vi "URG-04LX-UG01 Change Baud Rate.vi"(8 "error in":errorcluster, 10 "Baud Rate":u32, 11 "VISA Refnum in":refnum<visa-resource-name>) -> (0 "error out":errorcluster, 3 "VISA Refnum out":refnum<visa-resource-name>)   [LabVIEW 2018]
doc: "Changes the baud rate used to communicate with the URG-04LX-UG01."
uses:
  Type Definitions/Hokuyo Command Parameter.ctl
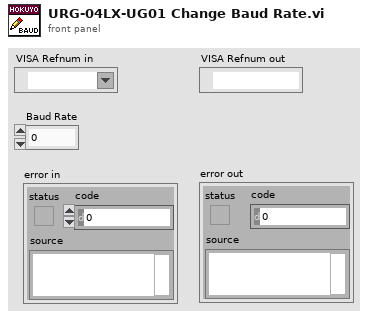
[diagram p1: front panel]
types:
  T1 = typedef "Hokuyo Command Parameter.ctl" = cluster{"Device Command":string, "String Characters":string}
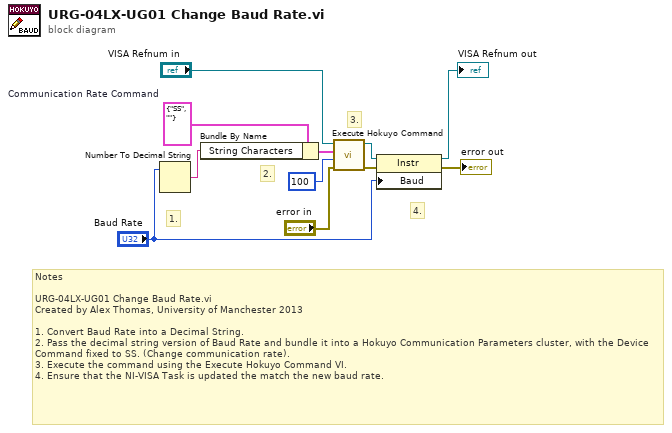
[diagram p0: block diagram]
diagram:
  w8 = T1 {"Device Command"="SS", "String Characters"=""}  # Communication Rate Command
  # "Notes\n\nURG-04LX-UG01 Change Baud Rate.vi\nCreated by Alex Thomas, University of Manchester 2013\n\n1. Convert Baud Rate into a Decimal String. \n2. Pass the decimal string version of Baud Rate and bundle it into a Hokuyo Communication Parameters cluster, with the Device Command fixed to SS. (Change communication rate).\n3. Execute the command using the Execute Hokuyo Command VI. \n4. Ensure that the NI-VISA Task is updated the match the new baud rate."
  # "4."
  # "3."
  # "2."
  # "1."
  n1 = Number To Decimal String(number="Baud Rate") -> (decimal integer string=w7:string)  [unwired: 1 in]
  n2 = Bundle By Name(cluster=w8, "String Characters"=w7) -> (w5:T1)
  n3 = call "Execute Hokuyo Command.vi"("error in (no error)"="error in", "milliseconds to wait"=u32 100, "Hokuyo Command Parameter"=w5, "VISA Refnum in"="VISA Refnum in") -> ("error out"=w4:errorcluster, "VISA Refnum out"=w2:refnum<visa-resource-name>)  [unwired: 5 in, 1 out]
  n4 = property class="Instr"(reference=w2, error in=w4, "Baud"="Baud Rate") -> (reference out=→"VISA Refnum out":refnum<visa-resource-name>, error out=→"error out":errorcluster)
